vi "Upload.vi"(8 "error in":errorcluster, 9 "Multiplexer":cluster{"Index":u16, "Sub-Index":u8} {"Index" format="%04x"; "Sub-Index" format="%02x"}, 10 "Node-ID":u8, 11 "CANopen Master in":refnum<class "CANopen Master.lvclass">) -> (0 "error out":errorcluster, 1 "Value":u8[](array[numeric]), 2 "Success?":bool, 3 "CANopen Master out":refnum<class "CANopen Master.lvclass">)   [LabVIEW 2024, in "CANopen Master.lvlib" / "CANopen Master.lvclass"]
uses:
  CANopen Master.lvclass
  CANopen Master.lvclass/CANopen Master.ctl
  SDO Manager/SDO Manager.lvclass
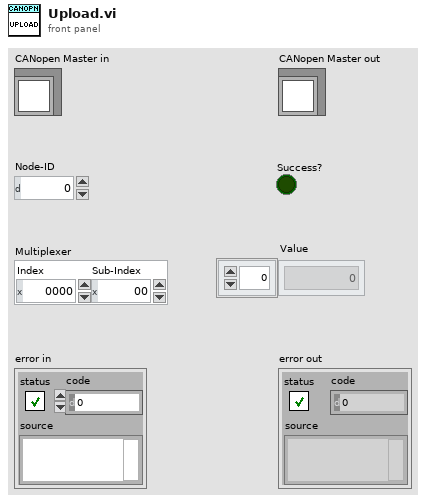
[diagram p1: front panel]
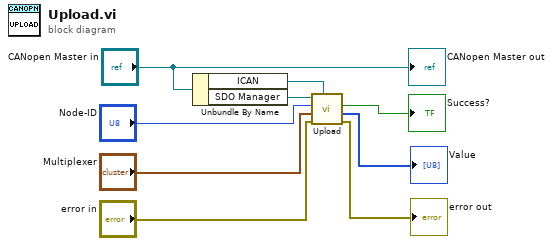
[diagram p0: block diagram]
diagram:
  n1 = Unbundle By Name("CANopen Master in") -> ("ICAN"=w7:refnum<class "ICAN.lvclass">, "SDO Manager"=w8:refnum<class "SDO Manager.lvclass">)
  n2 = call "Upload.vi"("ICAN"=w7, "Error In"="error in", "Multiplexer"="Multiplexer", "Node-ID"="Node-ID", "reference in"=w8) -> ("Error Out"=→"error out":errorcluster, "Value"=→"Value":u8[], "Success?"=→"Success?":bool)  [unwired: 3 in, 1 out]
  "CANopen Master out" <- "CANopen Master in"
